vi "Serialize.vi"(6 "priority":i32, 8 "error in (no error)":errorcluster, 11 "Serializable Message in":refnum<class "Serializable Msg.lvclass">) -> (0 "error out":errorcluster, 2 "Serialized Message":string)   [LabVIEW 2020, in "Serializer.lvlib" / "Serializable Message.lvlib" / "Serializable Msg.lvclass"]
uses:
  Serializable Msg.lvclass
  Serializable Msg.lvclass/Serializable Msg.ctl
  <vilib>/Utility/LVClass/Get LV Class Name.vi
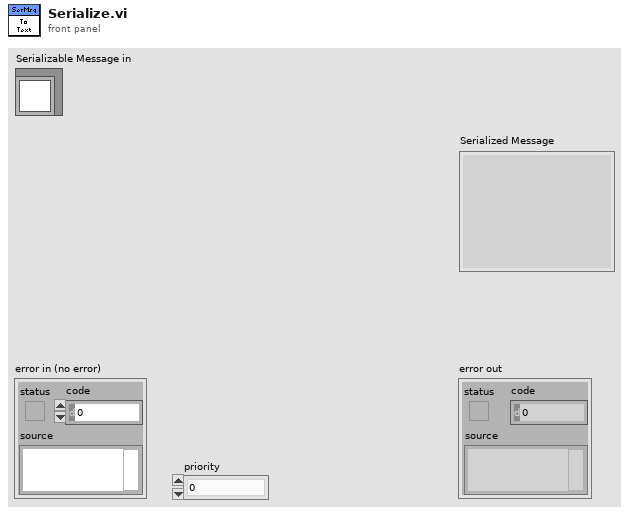
[diagram p1: front panel]
types:
  T1 = cluster{"Class name":string, "Priority":i32, "Data":string}
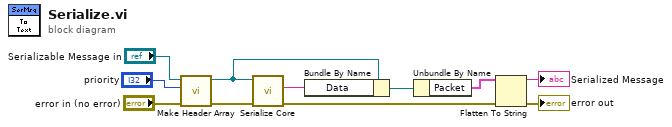
[diagram p0: block diagram]
diagram:
  n1 = call "Make Header Array.vi"("error in (no error)"="error in (no error)", "priority"="priority", "Serializable Msg in"="Serializable Message in") -> ("error out"=w2:errorcluster, "Serializable Msg out"=w4:refnum<class "Serializable Msg.lvclass">)  [unwired: 7 in]
  n2 = call-dynamic "Serialize Core.vi"("error in (no error)"=w2, "Serializable Message in"=w4) -> ("error out"=w1:errorcluster, "Serialized Message"=w9:string)  [unwired: 8 in]
  n3 = Bundle By Name(cluster=w4, "Data"=w9) -> (w7:refnum<class "Serializable Msg.lvclass">)
  n4 = Unbundle By Name(w7) -> ("Packet"=w6:T1)
  n5 = Flatten To String(anything=w6, error in (no error)=w1) -> (data string=→"Serialized Message":string, error out=→"error out":errorcluster)  [unwired: 2 in, 1 out]
